vi "Acquire.vi"(6 "UI":refnum<queue>, 8 "error in (no error)":errorcluster, 9 "Data Queue":refnum<queue>, 10 "Data Notifier":refnum<notifier>, 11 "Hardware Resources in":T1={"VISA resource name"="", "Mode (0: Normal) "=0, "Voltage"={"Element (0: All)"=0, "V Range (200)"=4}, "Current"={"A Range (2)"=7, "A Terminal (0: 5A)"=0, "Element (0: ALL)"=0}, "Observation Time"=10, "Modules on/off"={"Module 1"=FALSE, "Module 2"=FALSE, "Module 3"=FALSE, "Module 4"=FALSE}} {"Observation Time" items=["1ksec", "400sec", "200sec", "100sec", "40sec", "20sec", "10sec", "4sec", "2sec", "1sec", "400msec", "200msec", "100msec", "40msec", "20msec", "10msec", "4msec", "2msec", "1msec", "400usec", "200usec", "100usec", "40usec", "20usec", "10usec"]; "Mode (0: Normal)" items=["Normal", "Harmonics"]; "Current"."Element (0: ALL)" items=["All", "Element 1", "Element 2", "Element 3", "Element 4"]; "Current"."A Terminal (0: 5A)" items=["5A", "20A", "Sensor"]; "Current"."A Range (2)" items=["AUTO", "0.1", "0.2", "0.4", "1", "2", "4", "10", "20", "40", "100"]; "Voltage"."V Range (200)" items=["AUTO", "30", "60", "120", "200", "300", "600", "1200", "2000"]; "Voltage"."Element (0: All)" items=["All", "Element 1", "Element 2", "Element 3", "Element 4"]}) -> (0 "error out":errorcluster, 3 "Hardware Resources out":T1={"VISA resource name"="", "Mode (0: Normal) "=0, "Voltage"={"Element (0: All)"=0, "V Range (200)"=4}, "Current"={"A Range (2)"=7, "A Terminal (0: 5A)"=0, "Element (0: ALL)"=0}, "Observation Time"=10, "Modules on/off"={"Module 1"=FALSE, "Module 2"=FALSE, "Module 3"=FALSE, "Module 4"=FALSE}} {"Observation Time" items=["1ksec", "400sec", "200sec", "100sec", "40sec", "20sec", "10sec", "4sec", "2sec", "1sec", "400msec", "200msec", "100msec", "40msec", "20msec", "10msec", "4msec", "2msec", "1msec", "400usec", "200usec", "100usec", "40usec", "20usec", "10usec"]; "Mode (0: Normal)" items=["Normal", "Harmonics"]; "Current"."Element (0: ALL)" items=["All", "Element 1", "Element 2", "Element 3", "Element 4"]; "Current"."A Terminal (0: 5A)" items=["5A", "20A", "Sensor"]; "Current"."A Range (2)" items=["AUTO", "0.1", "0.2", "0.4", "1", "2", "4", "10", "20", "40", "100"]; "Voltage"."V Range (200)" items=["AUTO", "30", "60", "120", "200", "300", "600", "1200", "2000"]; "Voltage"."Element (0: All)" items=["All", "Element 1", "Element 2", "Element 3", "Element 4"]})   [LabVIEW 2014, in "Yokogawa.lvlib" / "YKPZ400 Acquisition.lvlib"]
doc: "Perform the acquisition. Replace the contents of this diagram with calls to acquisition hardware."
uses:
  YKPZ400 Acquisition.lvlib
  Hardware Configuration.ctl
  controls/electrical2.ctl
  support/Message Queue/Message Cluster.ctl
  support/Message Queue/Enqueue Message (Single).vi
  support/Message Queue/YKPZ400 Message Queue.lvlib
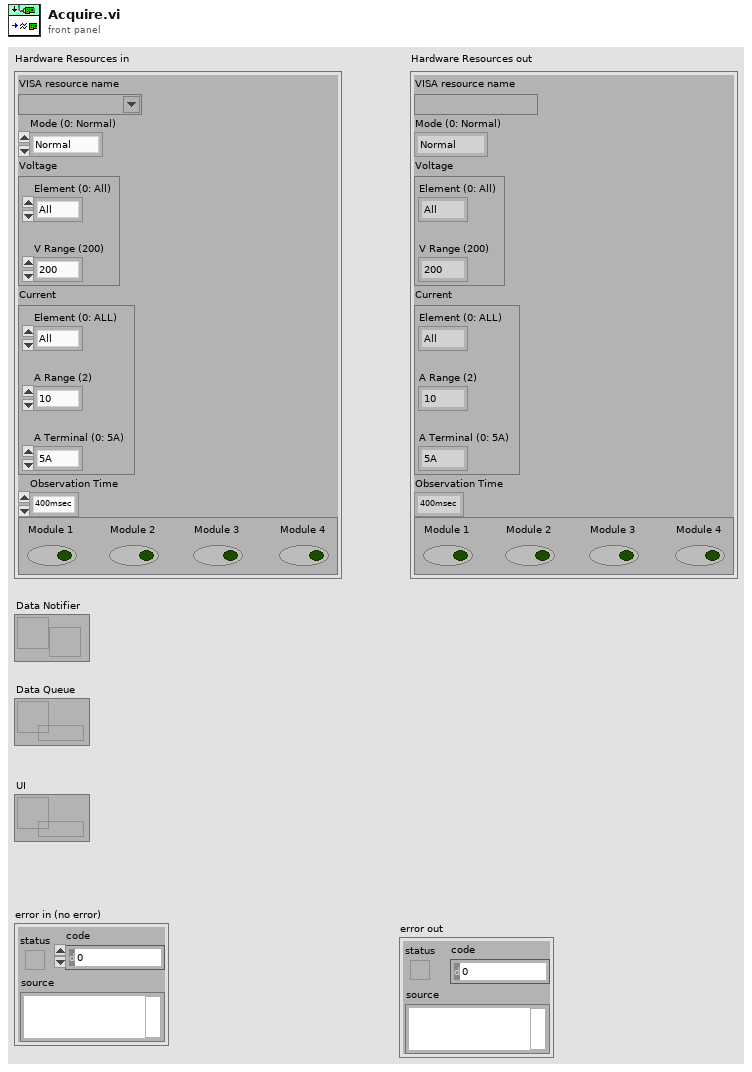
[diagram p1: front panel]
types:
  T1 = typedef "Yokogawa.lvlib/YKPZ400 Acquisition.lvlib/Hardware Configuration.ctl" = cluster{"VISA resource name":refnum<visa-resource-name>, "Mode (0: Normal) ":u16, "Voltage":cluster{"Element (0: All)":u16, "V Range (200)":u16}, "Current":cluster{"A Range (2)":u16, "A Terminal (0: 5A)":u16, "Element (0: ALL)":u16}, "Observation Time":u16, "Modules on/off":cluster{"Module 1":bool, "Module 2":bool, "Module 3":bool, "Module 4":bool}}
  T2 = typedef "Yokogawa.lvlib/YKPZ400 Acquisition.lvlib/electrical2.ctl" = cluster{"Time Stamp":timestamp, "Temperature (C)":dbl, "Electrical Data":string[][], "Waveform Graph":waveform(dbl)[]}
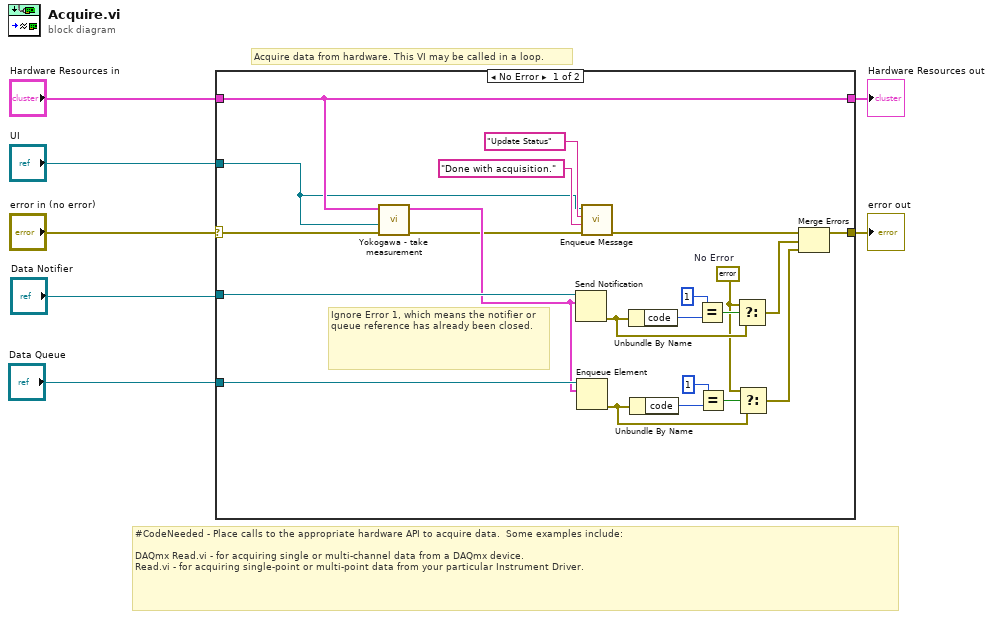
[diagram p0: block diagram]
diagram:
  # "Acquire data from hardware. This VI may be called in a loop."
  # "#CodeNeeded - Place calls to the appropriate hardware API to acquire data.  Some examples include:\n\nDAQmx Read.vi - for acquiring single or multi-channel data from a DAQmx device.\nRead.vi - for acquiring single-point or multi-point data from your particular Instrument Driver."
  n1 = case shown="No Error" "error in (no error)" {
    selector: "error in (no error)" -> [w15 w30]
    tunnel: [w29 w30] -> w6
    tunnel: "Hardware Resources in" -> [w14 w31]
    tunnel: [w14 w31] -> w4
    tunnel: "Data Notifier" -> [w28 _]
    tunnel: "Data Queue" -> [w17 _]
    tunnel: "UI" -> [w8 _]
    frame No Error {
      w16 = errorcluster {"status"=FALSE, "code"=0, "source"=""}  # No Error
      # "Ignore Error 1, which means the notifier or queue reference has already been closed."
      n2 = call "Yokogawa - take measurement.vi"("error in"=w15, "UI"=w8, "Hardware Resources in"=w14) -> ("error out"=w11:errorcluster, "Electrical Data 3"=w13:T2)  [unwired: 7 in]
      n3 = Send Notification(notification=w13, notifier=w28) -> (error out=w24:errorcluster)  [unwired: 1 in, 1 out]
      n4 = Enqueue Element(queue=w17, element=w13) -> (error out=w22:errorcluster)  [unwired: 2 in, 2 out]
      n5 = call-poly "Enqueue Message.vi"("error in (no error)"=w11, "Message Data"="Done with acquisition." ("Message"), "Message"="Update Status", "Message Queue"=w8) -> ("error out"=w10:errorcluster)  [unwired: 6 in, 1 out]
      n6 = Unbundle By Name(w24) -> ("code"=w27:i32)
      n7 = Unbundle By Name(w22) -> ("code"=w19:i32)
      n8 = Equal?(x=1, y=w27) -> (x = y?=w25:bool)
      n9 = Equal?(x=1, y=w19) -> (x = y?=w21:bool)
      n10 = Select(t=w16, s=w25, f=w24) -> (s? t:f=w23:errorcluster)
      n11 = Select(t=w16, s=w21, f=w22) -> (s? t:f=w18:errorcluster)
      n12 = Merge Errors(w10, w23, w18) -> (w29:errorcluster)
    }
    frame Error {
    }
  }
  "Hardware Resources out" <- w4
  "error out" <- w6
